vi "EncoderSafety.vi"(10 "Motor Velocity":dbl, 11 "Motor Current":dbl) -> (2 "Encoder_Dead?":bool)   [LabVIEW 2019]
uses:
  <vilib>/Rock Robotics/WPI/DriverStation/WPI_DriverStationRobotMode2.ctl
  mOS_XIII/MoS_XIII/Robot Global Data.vi
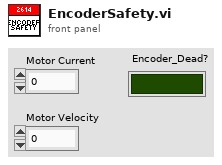
[diagram p1: front panel]
types:
  T1 = typedef "WPI_DriverStationRobotMode2.ctl" = enum16{"Autonomous Disabled", "Autonomous Enabled", "Teleop Disabled", "Teleop Enabled", "Disconnected", "Finish", "Test Disabled", "Test Enabled", "Emergency Stopped"}
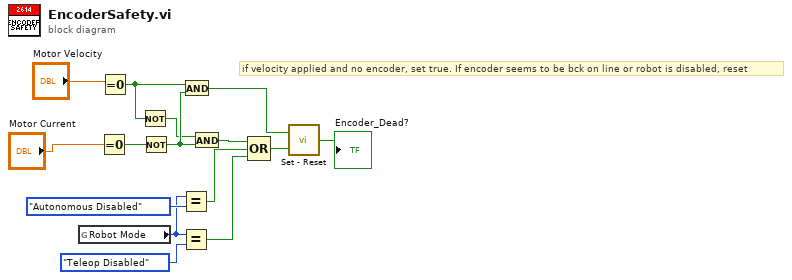
[diagram p0: block diagram]
diagram:
  # "if velocity applied and no encoder, set true. If encoder seems to be bck on line or robot is disabled, reset"
  n1 = global read "Robot Global Data.vi" "Robot Mode"() -> (w13:T1)
  n2 = Equal To 0?(x="Motor Current") -> (x = 0?=w15:bool)
  n3 = Equal To 0?(x="Motor Velocity") -> (x = 0?=w6:bool)
  n4 = Not(x=w6) -> (.not. x?=w7:bool)
  n5 = Not(x=w15) -> (.not. x?=w8:bool)
  n6 = Equal?(x=w13, y=WPI_DriverStationRobotMode2."Autonomous Disabled" ("Robot Mode")) -> (x = y?=w9:bool)
  n7 = Equal?(x=w13, y=WPI_DriverStationRobotMode2."Teleop Disabled" ("Robot Mode")) -> (x = y?=w10:bool)
  n8 = And(x=w6, y=w8) -> (x .and. y?=w12:bool)
  n9 = And(x=w7, y=w8) -> (x .and. y?=w5:bool)
  n10 = Compound Arithmetic op=OR(w5, w9, w10) -> (w4:bool)
  n11 = call "Set - Reset.vi"("Reset"=w4, "Set"=w12) -> ("Output"=→"Encoder_Dead?":bool)
